vi "Get Acquisition Registers.vi"(2 "acq":refnum<class "niUSRP Rx DSP v2 FPGA.lvclass">=refnum) -> (4 "acq registers":refnum<class "Address Space Collection.lvclass">)   [LabVIEW 2023]
uses:
  <instrlib>/niUSRP/Reference FPGA/Rx DSP/niUSRP Rx DSP v2 FPGA.lvclass
  <instrlib>/_niInstr/Instruction Framework/v1/FPGA/Interfaces/Address Space Collection/Address Space Collection.lvclass
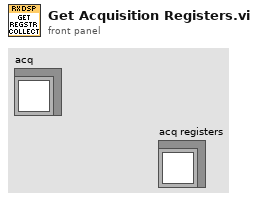
[diagram p1: front panel]
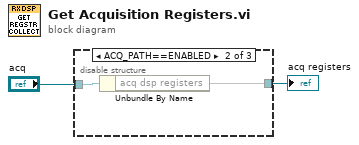
[diagram p0: block diagram]
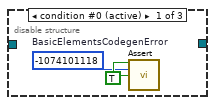
[diagram p2: hidden frame]
diagram:
  n1 = disable-structure shown="ACQ_PATH==ENABLED" {
    disable-tunnel: "acq" -> [_ w6 _]
    disable-tunnel: [_ w5 _] -> w1
    frame condition #0 (active) {
      w4 = TRUE ("assert")
      w3 = -1074101118  # BasicElementsCodegenError
      n2 = call <instrlib>:"Assert.vi"("assert"=w4, "error code"=w3, "enable show error"=w4) -> ()  [unwired: 13 in]
    }
    frame condition #1 {
      n3 = Unbundle By Name(w6) -> ("acq dsp registers"=w5)
    }
    frame condition #2 {
    }
  }
  "acq registers" <- w1
